vi "Determine Listbox Values.vi"(8 "error in (no error)":errorcluster, 10 "List of Objects":string[](array[string]), 11 "Section Ref in":T1 format="%.0x") -> (0 "error out":errorcluster, 1 "not present item indexes":i32[](array[numeric]), 2 "listbox text":string[][](array[string]), 3 "Section Ref out":T1 format="%.0x", 4 "reserved item indexes":i32[](array[numeric]))   [LabVIEW 2016, in "FPGA Addon System Explorer.lvlib"]
uses:
  FPGA Addon System Explorer.lvlib
  <vilib>/NI Veristand/Custom Device API/Custom Device Item Ref.ctl
  Shared/Constants.vi
  <vilib>/NI Veristand/Custom Device API/Get Item Property (String).vi
  <vilib>/NI Veristand/Custom Device API/Get Item Property (Dependent Node Pointer).vi
  <vilib>/NI VeriStand/Custom Device API/Custom Device API.lvlib
  Shared/FPGA Addon Shared.lvlib
  VeriStand-FPGA-Resource-Manager/Source/FPGA Resource Manager System Definition.lvlib
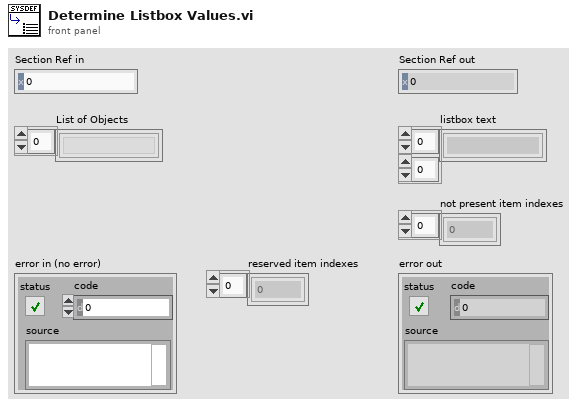
[diagram p1: front panel]
types:
  T1 = typedef "Custom Device API.lvlib/Custom Device Item Ref.ctl" = u64
  T2 = typedef "Custom Device API.lvlib/Custom Device Item Info.ctl" = cluster{"Name":string, "Is Channel":bool, "GUID":string, "Is Waveform":bool}
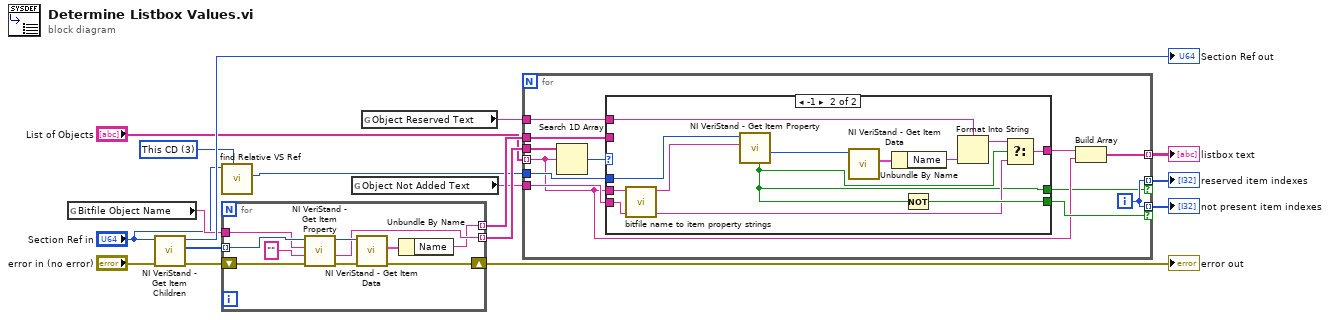
[diagram p0: block diagram]
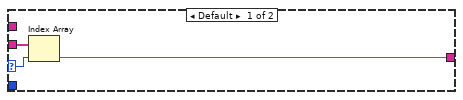
[diagram p2: hidden frame]
diagram:
  w4 = u16 3 items=["Targets", "Controller", "Custom Devices", "This CD", "This CD/Group", "This CD/Group/SubGroup"] ("Relative Type")
  n1 = global read "Constants.vi" "Bitfile Object Name"() -> (w7:string)
  n2 = call <vilib>:"NI VeriStand - Get Item Children.vi"("error in (no error)"="error in (no error)", "Item Ref in"="Section Ref in") -> ("error out"=w16:errorcluster, "Child Refs"=w15:T1[], "Item Ref out"=→"Section Ref out":T1)  [unwired: 6 in, 1 out]
  n3 = call "find Relative VS Ref.vi"("Relative Type"=w4, "Item Ref in"="Section Ref in") -> ("Relative Item Ref Out"=w3:T1)  [unwired: 5 in, 4 out]
  n4 = for {
    shift-right: [w22] -> w13
    shift-left: w16 -> [w27]
    tunnel: w15 -> [w25] mode=indexing
    tunnel: w7 -> [w24]
    tunnel: [w19] -> w12 mode=indexing
    tunnel: [w18] -> w11 mode=indexing
    n5 = call-poly <vilib>:"NI VeriStand - Get Item Property.vi"("error in (no error)"=w27, "Default Value"="", "Property Name"=w24, "Item Ref in"=w25) -> ("error out"=w26:errorcluster, "Value"=w19:string, "Item Ref out"=w21:T1)  [unwired: 4 in, 1 out]
    n6 = call <vilib>:"NI VeriStand - Get Item Data.vi"("error in (no error)"=w26, "Item Ref in"=w21) -> ("error out"=w22:errorcluster, "Item Info"=w20:T2)  [unwired: 6 in, 2 out]
    n7 = Unbundle By Name(w20) -> ("Name"=w18:string)
  }
  "error out" <- w13
  n8 = global read "Constants.vi" "Object Not Added Text"() -> (w8:string)
  n9 = global read "Constants.vi" "Object Reserved Text"() -> (w2:string)
  n10 = for {
    tunnel: "List of Objects" -> [w31] mode=indexing
    tunnel: w12 -> [w39]
    tunnel: w11 -> [w37]
    tunnel: [w35] -> w10 mode=indexing
    tunnel: w8 -> [w34]
    tunnel: [w29] -> w9 mode=indexing if=w33
    tunnel: w3 -> [w32]
    tunnel: w2 -> [w30]
    tunnel: [w29] -> w1 mode=indexing if=w28
    i -> [w29]
    n11 = Search 1D Array(1D array=w39, element=w31) -> (index of element=w38:i32)  [unwired: 1 in]
    n12 = case shown="-1" w38 {
      selector: w38 -> [w41 _]
      tunnel: [w40 w50] -> w36
      tunnel: w37 -> [w42 _]
      tunnel: w34 -> [_ w51]
      tunnel: [_ w52] -> w33
      tunnel: w32 -> [_ w54]
      tunnel: w31 -> [_ w53]
      tunnel: w30 -> [_ w48]
      tunnel: [_ w44] -> w28
      frame Default {
        n13 = Index Array(array=w42, index=w41) -> (element=w40:string)
      }
      frame -1 {
        n14 = call "bitfile name to item property strings.vi"("Name in bitfile"=w53) -> ("Reservation String"=w49:string)  [unwired: 9 in, 1 out]
        n15 = call-poly <vilib>:"NI VeriStand - Get Item Property.vi"("Property Name"=w49, "Item Ref in"=w54) -> ("Dependent Node Ref"=w47:T1, "Found"=w44:bool)  [unwired: 6 in, 2 out]
        n16 = call <vilib>:"NI VeriStand - Get Item Data.vi"("Item Ref in"=w47) -> ("Item Info"=w46:T2)  [unwired: 7 in, 3 out]
        n17 = Unbundle By Name(w46) -> ("Name"=w45:string)
        n18 = Not(x=w44) -> (.not. x?=w52:bool)
        n19 = Format Into String(format string=w48, w45) -> (resulting string=w43:string)  [unwired: 2 in, 1 out]
        n20 = Select(t=w43, s=w44, f=w51) -> (s? t:f=w50:string)
      }
    }
    n21 = Build Array(w36, w31) -> (w35:string[])
  }
  "listbox text" <- w10
  "not present item indexes" <- w9
  "reserved item indexes" <- w1
